vi "MQTT_PubRec_Send.vi"(8 "error in (no error)":errorcluster, 10 "Message ID":u16=10 format="%x", 11 "connection ID":refnum<k5>) -> (0 "error out":errorcluster, 2 "PubRec Message":u8[](array[numeric]) format="%x", 3 "connection ID out":refnum<k5>)   [LabVIEW 2017, in "MQTT_Functions.lvlib"]
uses:
  MQTT_Functions.lvlib
  Controls/MessageType.ctl
  Controls/Retain_Flag.ctl
  Controls/DUP_Flag.ctl
  Controls/QoS.ctl
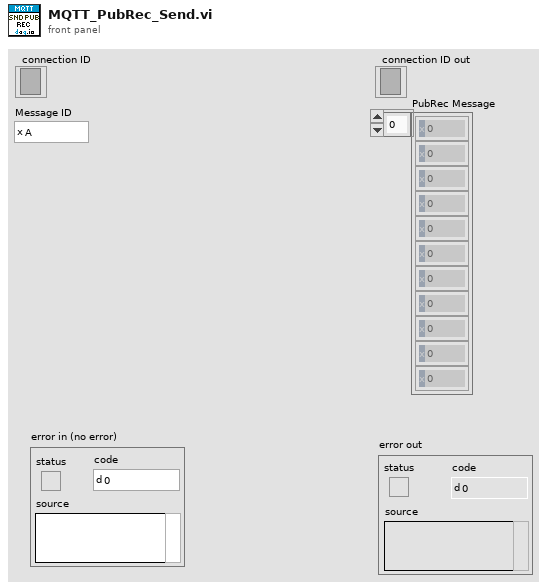
[diagram p1: front panel]
types:
  T1 = typedef "MQTT_Functions.lvlib/QoS.ctl" = enum8{"At most once", "At least once", "Exactly once", "Reserved"}
  T2 = typedef "MQTT_Functions.lvlib/DUP_Flag.ctl" = bool
  T3 = typedef "MQTT_Functions.lvlib/Retain_Flag.ctl" = bool
  T4 = typedef "MQTT_Functions.lvlib/MessageType.ctl" = enum32{"Reserved", "CONNECT", "CONNACK", "PUBLISH", "PUBACK", "PUBREC", "PUBREL", "PUBCOMP", "SUBSCRIBE", "SUBACK", "UNSUBSCRIBE", "UNSUBACK", "PINGREQ", "PINGRESP", "DISCONNECT", "Reserved2"}
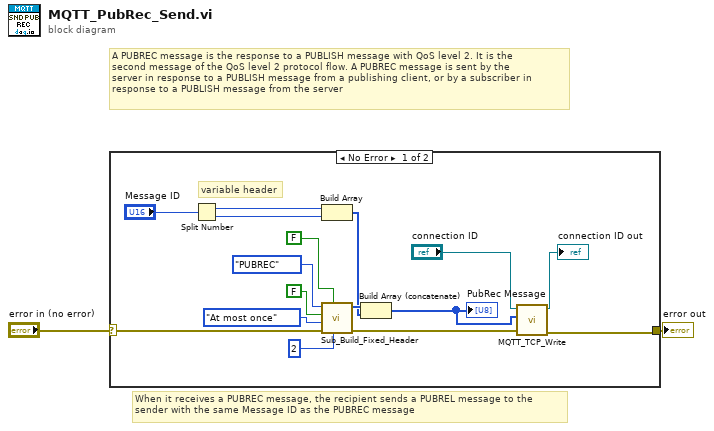
[diagram p0: block diagram]
diagram:
  # "When it receives a PUBREC message, the recipient sends a PUBREL message to the\nsender with the same Message ID as the PUBREC message"
  # "A PUBREC message is the response to a PUBLISH message with QoS level 2. It is the\nsecond message of the QoS level 2 protocol flow. A PUBREC message is sent by the\nserver in response to a PUBLISH message from a publishing client, or by a subscriber in\nresponse to a PUBLISH message from the server"
  n1 = case shown="No Error" "error in (no error)" {
    selector: "error in (no error)" -> [w9 w19]
    tunnel: [w5 w19] -> w1
    frame No Error {
      # "variable header"
      n2 = Split Number(x="Message ID") -> (hi(x)=w16:u8, lo(x)=w15:u8)
      n3 = Build Array(w16, w15) -> (w8:u8[])
      n4 = call "Sub_Build_Fixed_Header.vi"("Remaining Length"=u32 2, "Retain"=T3 FALSE, "error in (no error)"=w9, "QoS"=QoS."At most once", "DUP"=T2 FALSE, "MessageType"=MessageType."PUBREC") -> ("error out"=w6:errorcluster, "Fixed Header"=w17:u8[])  [unwired: 4 in]
      n5 = Build Array (concatenate)(w17, w8) -> (w7:u8[])
      "PubRec Message" <- w7
      n6 = call "MQTT_TCP_Write.vi"("error in (no error)"=w6, "data in"=w7, "connection ID"="connection ID") -> ("error out"=w5:errorcluster, "connection ID out"=→"connection ID out":refnum<k5>)  [unwired: 6 in, 1 out]
    }
    frame Error {
    }
  }
  "error out" <- w1
